vi "League Chat Parser.vi"() -> ()   [LabVIEW 2011]
uses:
  <vilib>/Utility/file.llb/Write To Spreadsheet File (string).vi
  <vilib>/Utility/file.llb/Read From Spreadsheet File (string).vi
panel:
  out "output cluster":T1
  out "concatenated string":string
  in  "Table Name":string="League_Data"
  in  "Victory or Defeat File":string(combo)="Victory"
  out "all rows":string[][](array[string])
  in  "Data Folder":path
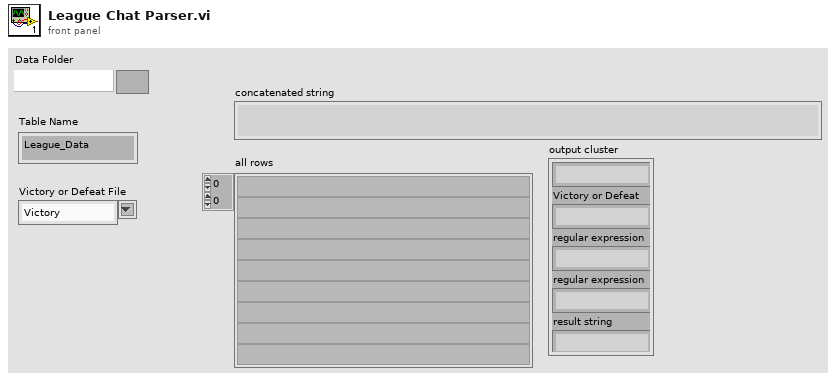
[diagram p1: front panel]
types:
  T1 = cluster{string, "Victory or Defeat":string, "regular expression":string, "regular expression":string, "result string":string, string, "result string":string}
  T2 = cluster{string, "Victory or Defeat File":string, "regular expression":string, "regular expression":string, "result string":string, string, "result string":string}
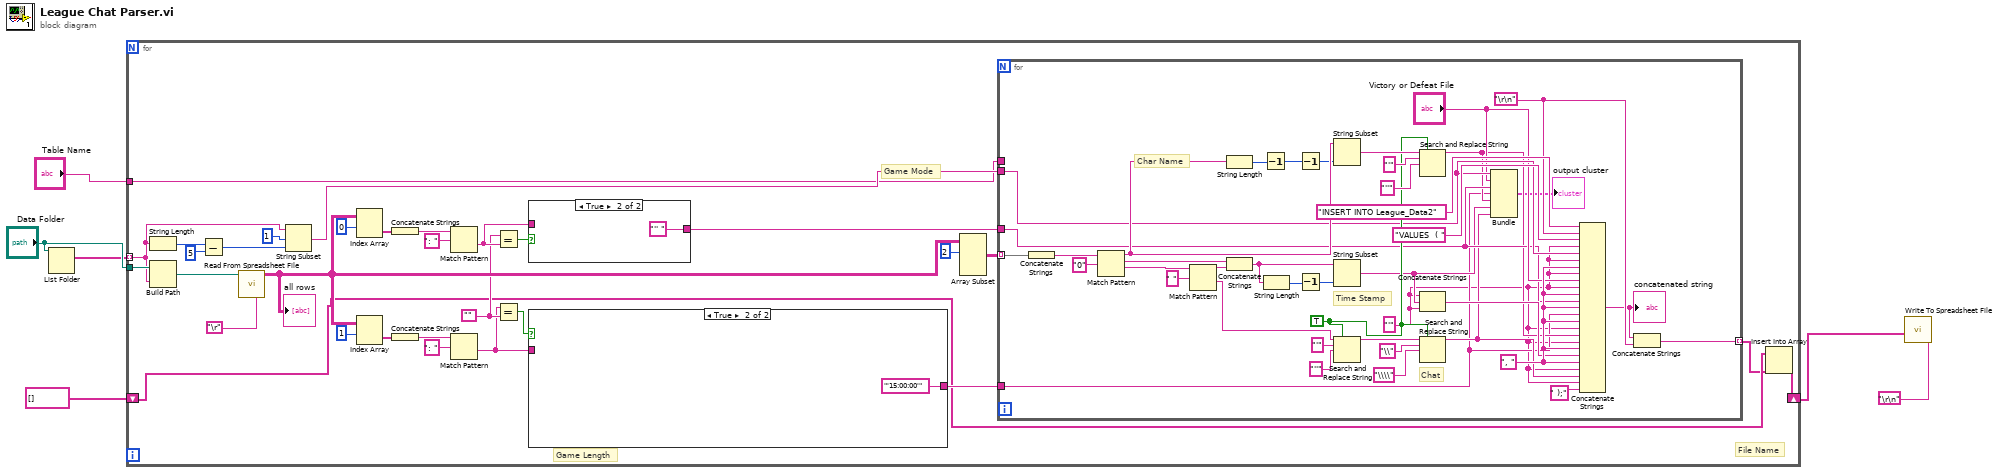
[diagram p0: block diagram]
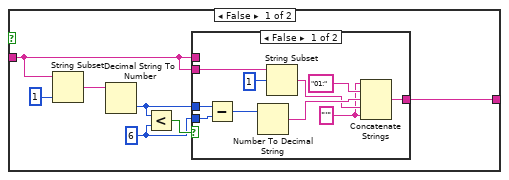
[diagram p2: hidden frame]
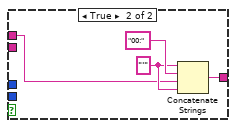
[diagram p3: hidden frame]
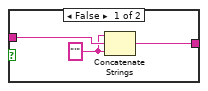
[diagram p4: hidden frame]
diagram:
  n1 = List Folder(path="Data Folder") -> (filenames=w5:string[])  [unwired: 3 in, 3 out]
  n2 = for {
    tunnel: "Data Folder" -> [w37]
    tunnel: w5 -> [w20] mode=indexing
    tunnel: "Table Name" -> [w17]
    shift-right: [w7] -> w2
    shift-left: string[] [] ("columns") -> [w9]
    w13 = ""
    # "Game Length"
    # "File Name"
    # "Game Mode"
    n3 = String Length(string=w20) -> (length=w23:i32)
    n4 = Build Path(base path=w37, name or relative path=w20) -> (appended path=w36:path)
    n5 = Subtract(x=w23, y=5) -> (x-y=w21:i32)
    n6 = call-poly <vilib>:"Read From Spreadsheet File.vi"("delimiter (\\t)"="\r", "file path (dialog if empty)"=w36) -> ("all rows"=w32:string[][])  [unwired: 5 in, 4 out]
    "all rows" <- w32
    n7 = String Subset(string=w20, offset (0)=1, length (rest)=w21) -> (substring=w19:string)
    n8 = Index Array(array=w32, index (row)=0) -> (element=w29:string[])  [unwired: 1 in]
    n9 = Index Array(array=w32, index (row)=1) -> (element=w24:string[])  [unwired: 1 in]
    n10 = Concatenate Strings(w29) -> (w28:string)
    n11 = Concatenate Strings(w24) -> (w26:string)
    n12 = Match Pattern(string=w28, regular expression=": ") -> (after substring=w14:string)  [unwired: 1 in, 3 out]
    n13 = Match Pattern(string=w26, regular expression=": ") -> (after substring=w11:string)  [unwired: 1 in, 3 out]
    n14 = Equal?(x=w13, y=w14) -> (x = y?=w16:bool)
    n15 = Equal?(x=w11, y=w13) -> (x = y?=w12:bool)
    n16 = case shown="True" w16 {
      tunnel: [w60 "'' " ("regular expression")] -> w15
      tunnel: w14 -> [w62 _]
      frame False {
        w61 = "'" ("string")
        n17 = Concatenate Strings(w61, w62, w61) -> (w60:string)
      }
      frame True {
      }
    }
    n18 = case shown="True" w12 {
      tunnel: [w44 "'15:00:00'" ("regular expression")] -> w10
      tunnel: w11 -> [w38 _]
      frame False {
        w39 = 6 ("y")
        n19 = String Subset(string=w38, length (rest)=1 ("length (rest)")) -> (substring=w42:string)  [unwired: 1 in]
        n20 = Decimal String To Number(string=w42) -> (number=w40:i32)  [unwired: 2 in, 1 out]
        n21 = Less?(x=w40, y=w39) -> (x < y?=w41:bool)
        n22 = case shown="False" w41 {
          tunnel: [w47 w57] -> w44
          tunnel: w38 -> [_ w55]
          tunnel: w40 -> [w54 _]
          tunnel: w39 -> [w53 _]
          tunnel: w38 -> [w51 _]
          frame False {
            w45 = "'" ("string")
            n23 = Subtract(x=w54, y=w53) -> (x-y=w50:i32)
            n24 = Number To Decimal String(number=w50) -> (decimal integer string=w49:string)  [unwired: 1 in]
            n25 = String Subset(string=w51, offset (0)=1) -> (substring=w48:string)  [unwired: 1 in]
            n26 = Concatenate Strings(w45, "01:" ("string"), w49, w48, w45) -> (w47:string)
          }
          frame True {
            w56 = "'" ("string")
            n27 = Concatenate Strings(w56, "00:" ("string"), w55, w56) -> (w57:string)
          }
        }
      }
      frame True {
      }
    }
    n28 = Array Subset(array=w32, index (row)=2) -> (w30:string[][])  [unwired: 3 in]
    n29 = for {
      tunnel: w30 -> [w103] mode=indexing
      tunnel: w19 -> [w74]
      tunnel: w15 -> [w72]
      tunnel: w10 -> [w67]
      tunnel: w17 -> [_]
      tunnel: [w64] -> w8 mode=indexing
      w76 = TRUE ("replace all? (F)")
      w86 = "\r\n"
      w89 = ", " ("string")
      w66 = "'"
      # "Time Stamp"
      # "Chat"
      # "Char Name"
      n30 = Concatenate Strings(w103) -> (w102:string)
      n31 = Match Pattern(string=w102, regular expression="0") -> (before substring=w99:string, match substring=w96:string, after substring=w95:string)  [unwired: 1 in, 1 out]
      n32 = Match Pattern(string=w95, regular expression=" ") -> (before substring=w93:string, after substring=w83:string)  [unwired: 1 in, 2 out]
      n33 = String Length(string=w99) -> (length=w100:i32)
      n34 = Concatenate Strings(w96, w93) -> (w91:string)
      n35 = Decrement(x=w100) -> (x-1=w98:i32)
      n36 = String Length(string=w91) -> (length=w92:i32)
      n37 = Decrement(x=w98) -> (x-1=w97:i32)
      n38 = Decrement(x=w92) -> (x-1=w90:i32)
      n39 = String Subset(string=w99, length (rest)=w97) -> (substring=w80:string)  [unwired: 1 in]
      n40 = String Subset(string=w91, length (rest)=w90) -> (substring=w70:string)  [unwired: 1 in]
      n41 = Search and Replace String(replace all?=w76, input string=w83, search string="'", replace string="''" ("replace string (\"\")")) -> (result string=w77:string)  [unwired: 4 in, 3 out]
      n42 = Search and Replace String(replace all?=w76, input string=w80, search string="'", replace string="''" ("replace string (\"\")")) -> (result string=w71:string)  [unwired: 4 in, 3 out]
      n43 = Concatenate Strings(w66, w70, w66) -> (w75:string)
      n44 = Search and Replace String(replace all?=w76, input string=w77, search string="\\", replace string="\\\\" ("replace string (\"\")")) -> (result string=w69:string)  [unwired: 4 in, 3 out]
      n45 = Bundle(w74, "Victory or Defeat File"="Victory or Defeat File", "regular expression"=w72, "regular expression"=w67, "result string"=w71, w70, "result string"=w69) -> (→"output cluster":T2)  [unwired: 1 in]
      n46 = Concatenate Strings("INSERT INTO League_Data2", w86, "VALUES  ( ", w66, w74, w66, w89, w66, "Victory or Defeat File", w66, w89, w72, w89, w67, w89, w66, w71, w66, w89, w75, w89, w66, w69, w66, " );" ("string")) -> (w68:string)
      "concatenated string" <- w68
      n47 = Concatenate Strings(w68, w86) -> (w64:string)
    }
    n48 = Insert Into Array(array=w9, new element=w8) -> (w7:string[])  [unwired: 1 in]
  }
  n49 = call-poly <vilib>:"Write To Spreadsheet File.vi"("delimiter (\\t)"="\r\n", "1D data"=w2) -> ()  [unwired: 6 in, 1 out]
